vi "PH_SRDG645.get Hardware Settings.vi"(0 "i ref in":refnum<vi>, 5 "error in":errorcluster) -> (14 "i ref out":refnum<vi>, 19 "error out":errorcluster)   [LabVIEW 2014, in "PH_SRDG645.lvlib"]
doc: "This VI queries all relevant hardware settings and writes it to own attributes and the GUI."
uses:
  PH_SRDG645.lvlib
  instr.lib/SRDG645/Driver/Channel.ctl
  instr.lib/SRDG645/Driver/Output BNC.ctl
  instr.lib/SRDG645/Stanford Research DG645 - Driver.lvlib
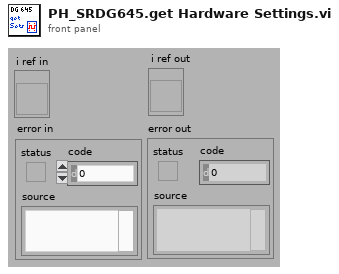
[diagram p1: front panel]
types:
  T1 = typedef "Stanford Research DG645 - Driver.lvlib/Output BNC.ctl" = i32
  T2 = typedef "Stanford Research DG645 - Driver.lvlib/Channel.ctl" = i32
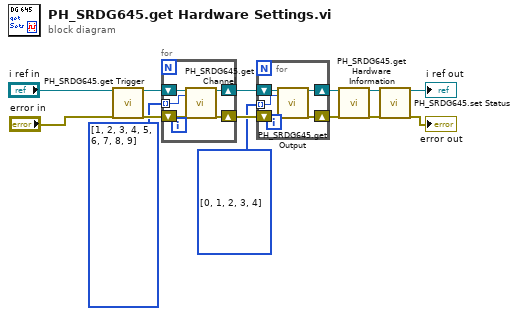
[diagram p0: block diagram]
diagram:
  w9 = T1[] [0, 1, 2, 3, 4] items=["T0", "AB", "CD", "EF", "GH"]
  w11 = T2[] [1, 2, 3, 4, 5, 6, 7, 8, 9] items=["T0", "T1", "A", "B", "C", "D", "E", "F", "G", "H"]
  n1 = call "PH_SRDG645.get Trigger.vi"("i ref in"="i ref in", "error IO"="error in") -> ("i ref out"=w12:refnum<vi>, "error out"=w14:errorcluster)  [unwired: 16 in]
  n2 = for {
    shift-right: [w16] -> w10
    shift-left: w12 -> [w17]
    shift-right: [w18] -> w13
    shift-left: w14 -> [w19]
    tunnel: w11 -> [w15] mode=indexing
    n3 = call "PH_SRDG645.get Channel.vi"("i ref in"=w17, "Channel (T0)"=w15, "error IO"=w19) -> ("i ref out"=w16:refnum<vi>, "error out"=w18:errorcluster)  [unwired: 15 in]
  }
  n4 = for {
    shift-right: [w21] -> w2
    shift-left: w10 -> [w22]
    shift-right: [w23] -> w1
    shift-left: w13 -> [w24]
    tunnel: w9 -> [w20] mode=indexing
    n5 = call "PH_SRDG645.get Output.vi"("i ref in"=w22, "Output BNC (T0)"=w20, "error IO"=w24) -> ("i ref out"=w21:refnum<vi>, "error out"=w23:errorcluster)  [unwired: 15 in]
  }
  n6 = call "PH_SRDG645.get Hardware Information.vi"("i ref in"=w2, "error in"=w1) -> ("i ref out"=w6:refnum<vi>, "error out"=w4:errorcluster)  [unwired: 16 in]
  n7 = call "PH_SRDG645.set Status.vi"("i ref in"=w6, "error in"=w4) -> ("i ref out"=→"i ref out":refnum<vi>, "error out"=→"error out":errorcluster)  [unwired: 16 in]
